vi "Nonlinearity Correction.vi"(8 "error in (no error)":errorcluster, 9 "Dark Spectrum":dbl[](array[numeric]), 10 "Spectrum by Pixels":dbl[](array[numeric]), 11 "VISA resource name":refnum<visa-resource-name>) -> (0 "error out":errorcluster, 2 "Spectrum by Pixels Linearized":dbl[](array[numeric]), 3 "VISA resource name out":refnum<visa-resource-name>)   [LabVIEW 2013, in "Ocean Optics 2000 4000.lvlib"]
doc: "Applies non-linearity correction to the spectrum. If a dark spectrum is provided it is first subtracted off then the correction is applied then the dark spectrum is added back in. If no dark spectrum is supplied then the correction is directly applied. This is equivalent to providing a dark spectrum of all zeros."
uses:
  <instrlib>/Ocean Optics 2000 4000/Ocean Optics 2000 4000.lvlib
  <vilib>/Analysis/polynomials.llb/1D Polynomial Evaluation (DBL).vi
  <vilib>/Analysis/NI_AALPro.lvlib
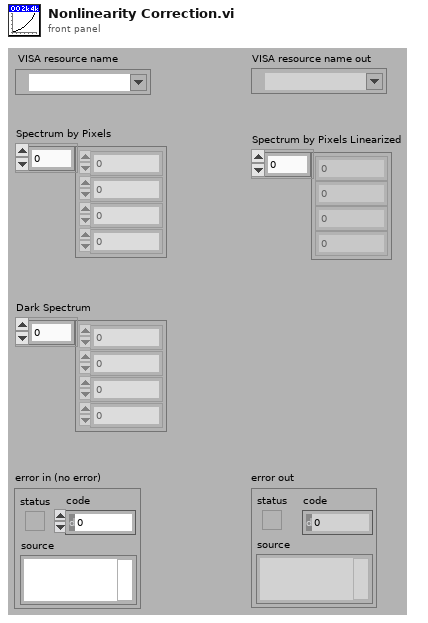
[diagram p1: front panel]
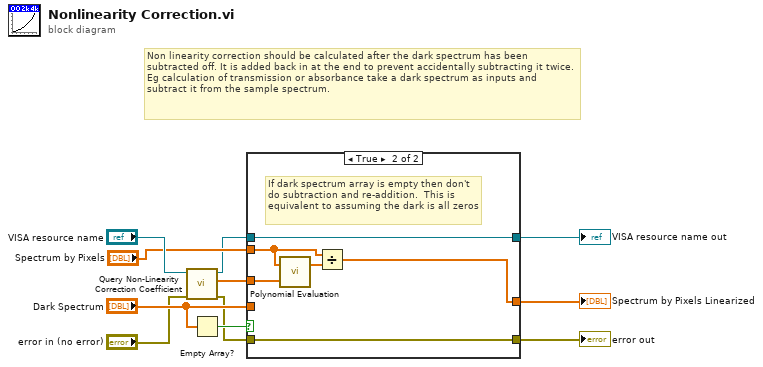
[diagram p0: block diagram]
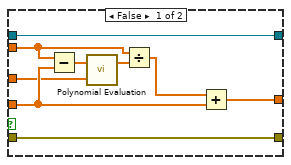
[diagram p2: hidden frame]
diagram:
  # "Non linearity correction should be calculated after the dark spectrum has been subtracted off. It is added back in at the end to prevent accidentally subtracting it twice.  Eg calculation of transmission or absorbance take a dark spectrum as inputs and subtract it from the sample spectrum."
  n1 = call <instrlib>:"Query Non-Linearity Correction Coefficient.vi"("error in (no error)"="error in (no error)", "VISA resource name"="VISA resource name") -> ("error out"=w2:errorcluster, "Non-Linearity Correction Coefficient"=w3:dbl[], "VISA resource name out"=w1:refnum<visa-resource-name>)  [unwired: 6 in, 1 out]
  n2 = Empty Array?(array="Dark Spectrum") -> (empty?=w4:bool)
  n3 = case shown="True" w4 {
    tunnel: w1 -> [w14 w25]
    tunnel: "Dark Spectrum" -> [w20 _]
    tunnel: [w19 w21] -> w6
    tunnel: w2 -> [w13 w24]
    tunnel: [w13 w24] -> w10
    tunnel: [w14 w25] -> w9
    tunnel: "Spectrum by Pixels" -> [w18 w23]
    tunnel: w3 -> [w12 w26]
    frame False {
      n4 = Subtract(x=w18, y=w20) -> (x-y=w15:dbl[])
      n5 = call-poly <vilib>:"Polynomial Evaluation.vi"("P(x)"=w12, "A"=w15) -> ("P(A)"=w17:dbl[])  [unwired: 1 out]
      n6 = Divide(x=w18, y=w17) -> (x/y=w16:dbl[])
      n7 = Add(x=w16, y=w20) -> (x+y=w19:dbl[])
    }
    frame True {
      # "If dark spectrum array is empty then don't do subtraction and re-addition.  This is equivalent to assuming the dark is all zeros"
      n8 = call-poly <vilib>:"Polynomial Evaluation.vi"("P(x)"=w26, "A"=w23) -> ("P(A)"=w22:dbl[])  [unwired: 1 out]
      n9 = Divide(x=w23, y=w22) -> (x/y=w21:dbl[])
    }
  }
  "Spectrum by Pixels Linearized" <- w6
  "VISA resource name out" <- w9
  "error out" <- w10
